vi "Close Panel.vi"(8 "error in (no error)":errorcluster, 11 "Panel Helper in":refnum<class "Panel Helper.lvclass">) -> (0 "error out":errorcluster)   [LabVIEW 2023, in "Panel Actor.lvlib" / "Panel.lvlib" / "Panel Helper.lvclass"]
uses:
  Panel Helper.lvclass
  Events.ctl
  Panel Helper.lvclass/Panel Helper.ctl
  Panel Registry/Panel Registry.lvclass
  Panel.lvlib
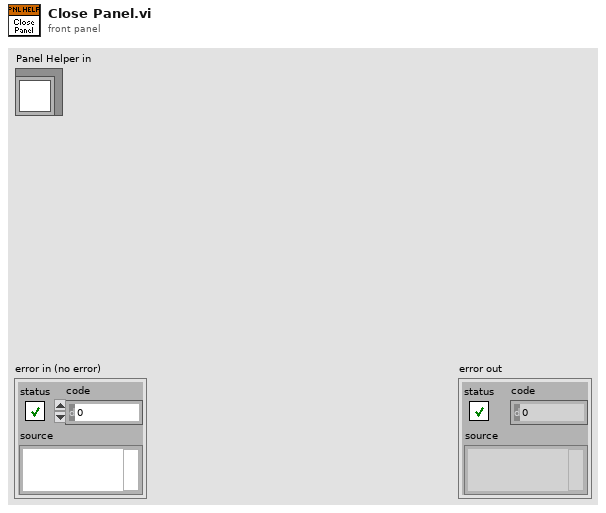
[diagram p1: front panel]
types:
  T1 = typedef "Panel Actor.lvlib/Panel.lvlib/Panel Helper.lvclass/Events.ctl" = enum16{"Initialized", "Shown", "Hidden", "Closed"}
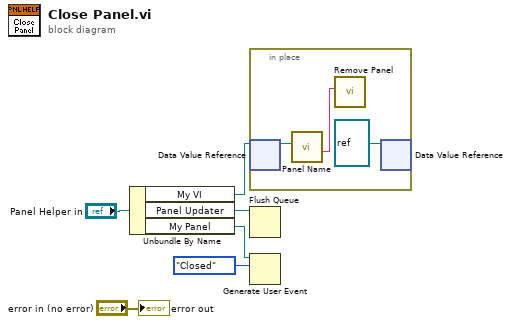
[diagram p0: block diagram]
diagram:
  n1 = Unbundle By Name("Panel Helper in") -> ("My VI"=w5:refnum<data-value>, "Panel Updater"=w4:refnum<queue>, "My Panel"=w2:refnum<user-event>)
  n2 = in-place {
    n3 = in-place-dvr #1(w5) -> (w8:refnum<vi>)  [unwired: 1 out]
    n4 = call "Panel Name.vi"("VI in"=w8) -> ("Name"=w7:string)  [unwired: 9 in, 1 out]
    n5 = call "Remove Panel.vi"("Panel"=w7) -> ()  [unwired: 10 in, 1 out]
    n6 = in-place-dvr #1(refnum<vi> refnum ("data value")) -> ()  [unwired: 2 out]
  }
  n7 = Flush Queue(queue=w4) -> ()  [unwired: 1 in, 3 out]
  n8 = Generate User Event(user event=w2, event data cluster=Events."Closed" ("event data")) -> ()  [unwired: 2 in, 2 out]
  "error out" <- "error in (no error)"
